vi "is_cmds_empty.vi"(8 "error in (no error)":errorcluster, 11 "OneMotion in":refnum<class "OneMotion.lvclass">) -> (0 "error out":errorcluster, 2 "cmds empty?":bool, 3 "OneMotion out":refnum<class "OneMotion.lvclass">)   [LabVIEW 2016, in "MotionControl_UFO_3DOF.lvlib" / "OneMotion.lvclass"]
uses:
  <userlib>/MotionControl_UFO_3DOF/OneMotion/OneMotion.lvclass
  <userlib>/MotionControl_UFO_3DOF/OneMotion/OneMotion.lvclass/OneMotion.ctl
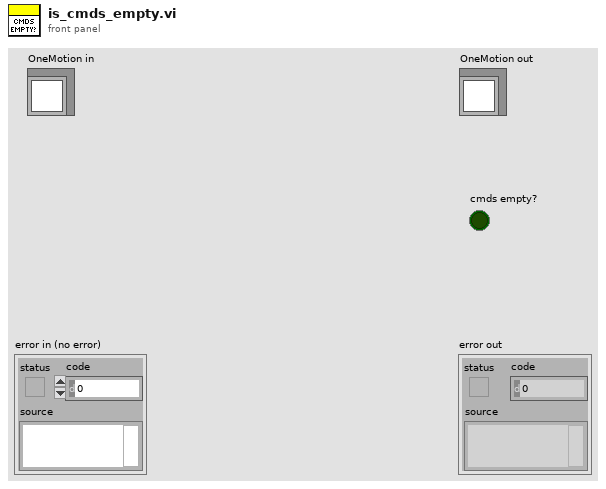
[diagram p1: front panel]
types:
  T1 = typedef "MotionControl_UFO_3DOF.lvlib/OneMotion.lvclass/cmd_motion.ctl" = enum16{"NONE", "MOVE_MOTION", "EXIT", "STP_MOTION", "SPEED_MOTION", "WAIT_FOR_S3", "WAIT_A_TIME", "SKIP", "RETRACT_BEFORE_ROT"}
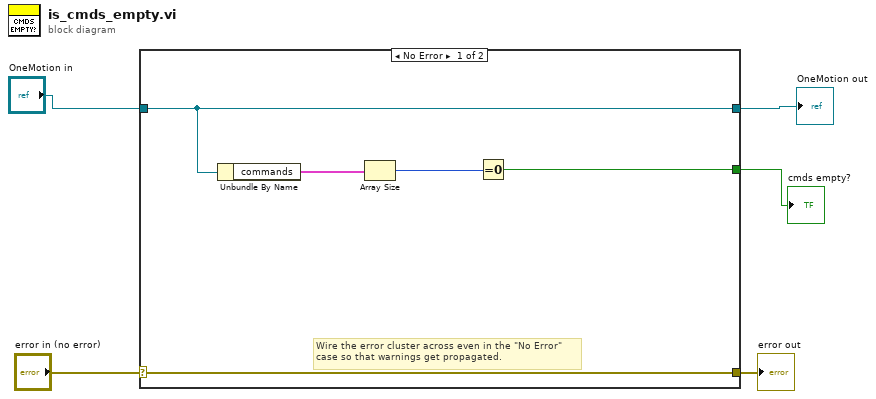
[diagram p0: block diagram]
diagram:
  n1 = case shown="No Error" "error in (no error)" {
    selector: "error in (no error)" -> [w10 w12]
    tunnel: [w10 w12] -> w4
    tunnel: [w9 w11] -> w1
    tunnel: "OneMotion in" -> [w9 w11]
    tunnel: [w6 _] -> w3
    frame No Error {
      # "Wire the error cluster across even in the \"No Error\"\ncase so that warnings get propagated."
      n2 = Unbundle By Name(w9) -> ("commands"=w8:cluster{"cmd":T1, "cmd data":variant}[])
      n3 = Array Size(array=w8) -> (size(s)=w7:i32)
      n4 = Equal To 0?(x=w7) -> (x = 0?=w6:bool)
    }
    frame Error {
    }
  }
  "error out" <- w4
  "cmds empty?" <- w3
  "OneMotion out" <- w1
